vi "Hub_Connect to Laser_Dx.vi"() -> ()   [LabVIEW 2020]
uses:
  Anemometry/Anemometry Sub Vis/Globals/LDA_global.vi
panel:
  out "reference out":refnum<k7>
  in  "BSALaserCtrl.IBSALaser 2":refnum<k7>
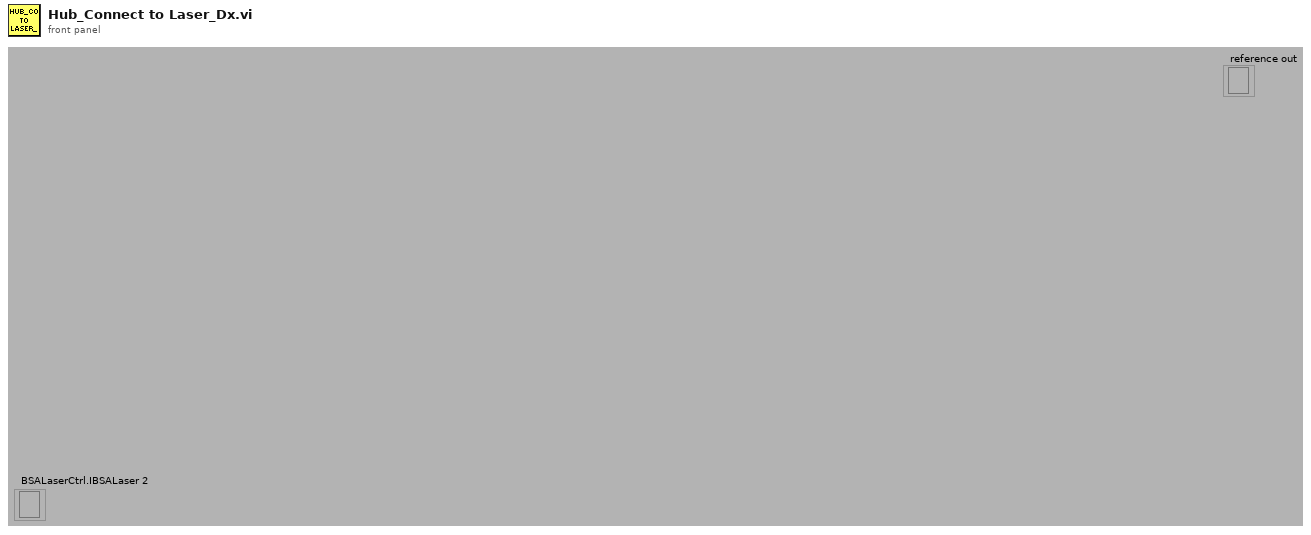
[diagram p1: front panel]
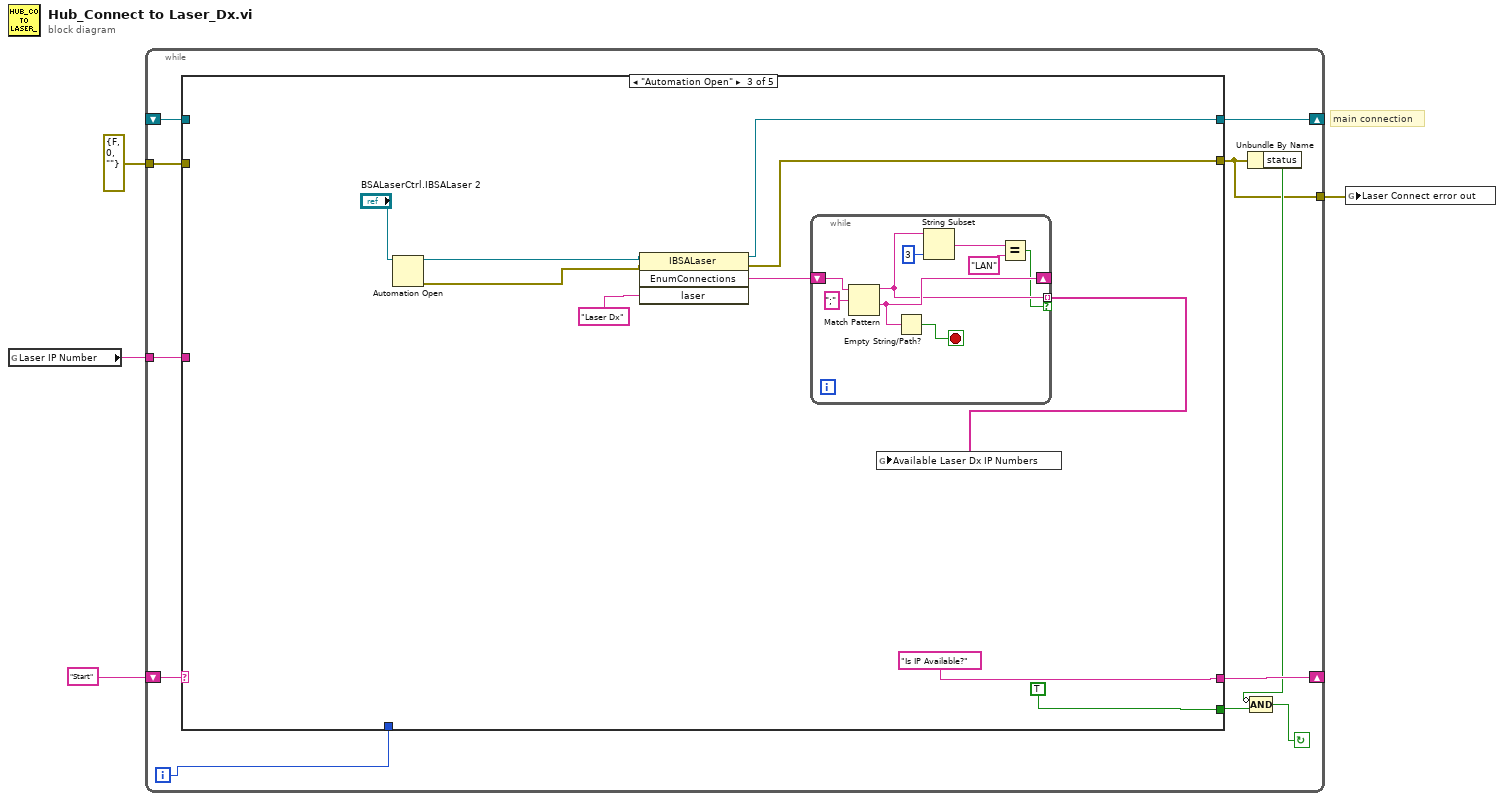
[diagram p0: block diagram]
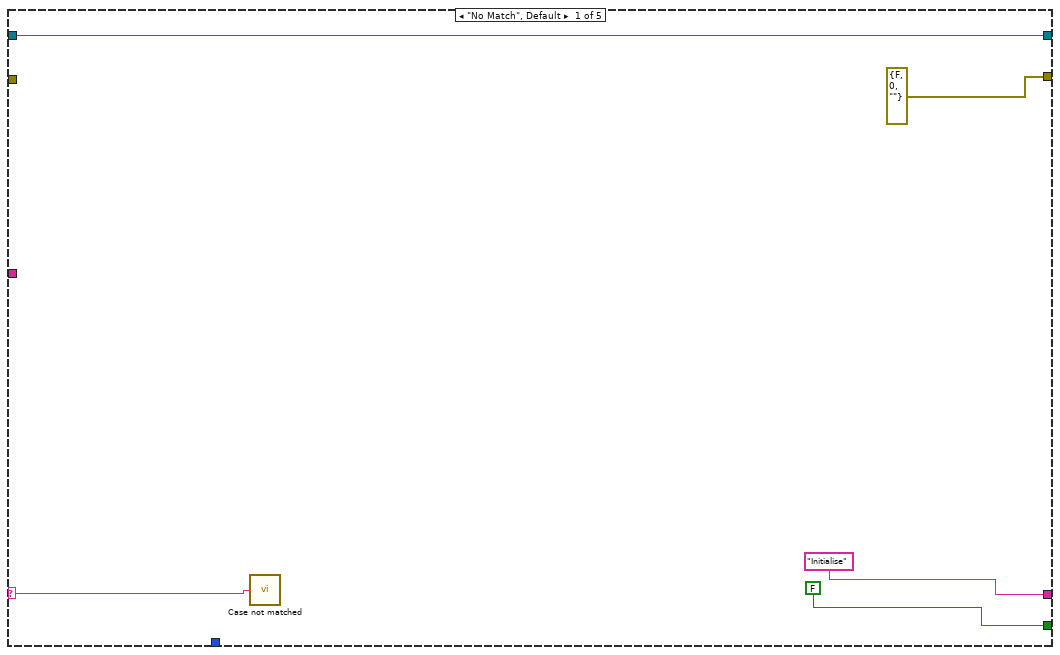
[diagram p2: hidden frame]
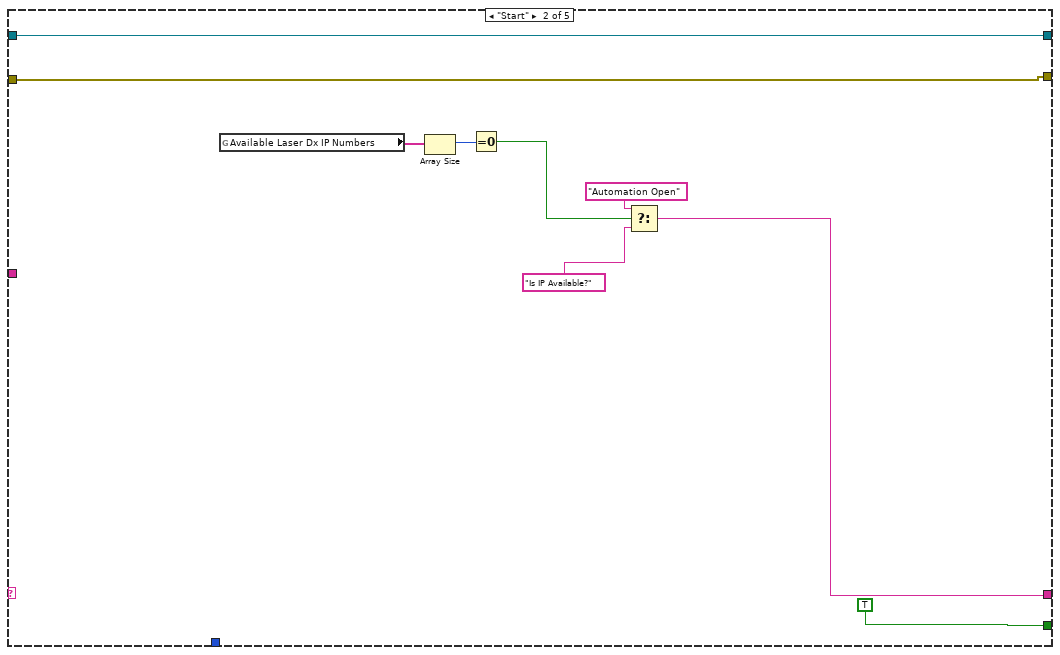
[diagram p3: hidden frame]
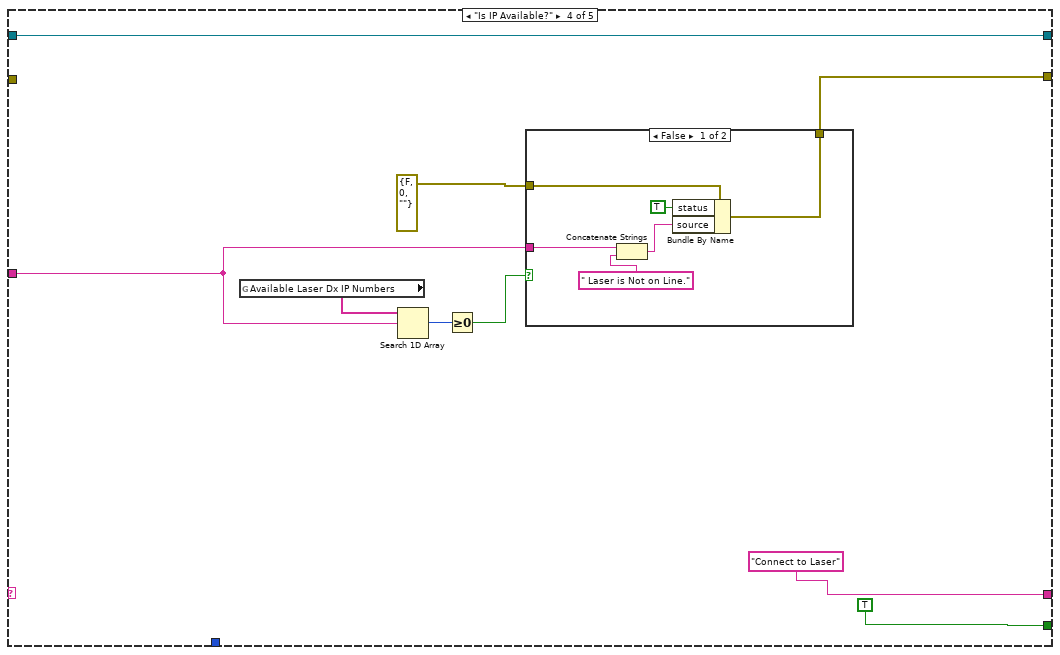
[diagram p4: hidden frame]
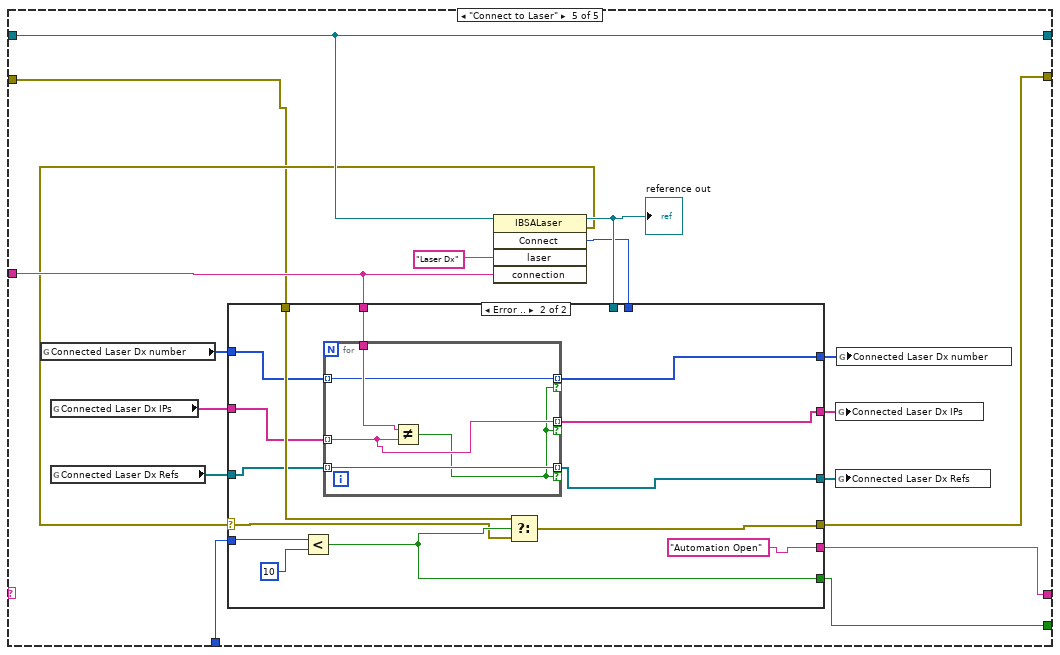
[diagram p6: hidden frame]
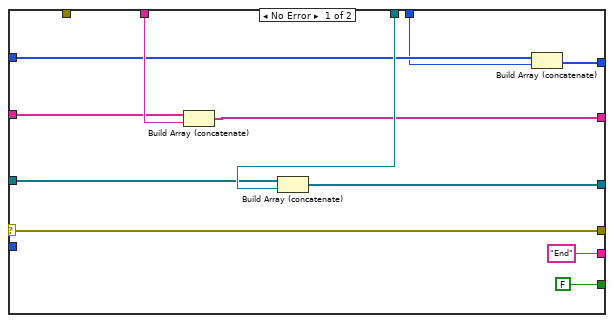
[diagram p7: hidden frame]
diagram:
  # "main connection"
  n1 = global read "LDA_global.vi" "Laser IP Number"() -> (w3:string)
  n2 = while {
    shift-left: "Start" -> [w14]
    shift-right: [w15] -> _
    shift-right: [w13] -> _
    shift-left: _ -> [w12]
    tunnel: w3 -> [w11]
    tunnel: [w7] -> w2
    tunnel: errorcluster {"status"=FALSE, "code"=0, "source"=""} ("error out") -> [w5]
    i -> [w6]
    stop <- w9 continue-if-true
    n3 = case shown="\"Automation Open\"" w14 {
      selector: w14 -> [w18 _ _ _ _]
      tunnel: [FALSE TRUE TRUE TRUE w74] -> w10
      tunnel: ["Initialise" w22 "Is IP Available?" "Connect to Laser" w73] -> w15
      tunnel: [w17 w26 w34 w54 w78] -> w13
      tunnel: w12 -> [w17 w26 _ w54 w78]
      tunnel: w11 -> [_ _ _ w49 w79]
      tunnel: [errorcluster {"status"=FALSE, "code"=0, "source"=""} ("error out") w21 w31 w52 w75] -> w7
      tunnel: w6 -> [_ _ _ _ w76]
      tunnel: w5 -> [_ w21 _ _ w72]
      frame "No Match", Default {
        n4 = call "Case not matched.vi"("Case Name not Matched"=w18) -> ()
      }
      frame "Start" {
        n5 = global read "LDA_global.vi" "Available Laser Dx IP Numbers"() -> (w28:string[])
        n6 = Array Size(array=w28) -> (size(s)=w27:i32)
        n7 = Equal To 0?(x=w27) -> (x = 0?=w25:bool)
        n8 = Select(t="Automation Open", s=w25, f="Is IP Available?") -> (s? t:f=w22:string)
      }
      frame "Automation Open" {
        n9 = Automation Open(Automation Refnum="BSALaserCtrl.IBSALaser 2") -> (Automation Refnum=w30:refnum<k7>, error out=w36:errorcluster)  [unwired: 3 in]
        n10 = invoke class="IBSALaser" method="EnumConnections"(reference=w30, error in=w36, "laser"="Laser Dx") -> (reference out=w34:refnum<k7>, error out=w31:errorcluster, "EnumConnections"=w38:string)  [unwired: 1 in, 1 out]
        n11 = while {
          shift-right: [w45] -> _
          shift-left: w38 -> [w47]
          tunnel: [w44] -> w33 mode=indexing if=w40
          stop <- w46 stop-if-true
          n12 = Match Pattern(string=w47, regular expression=";") -> (before substring=w44:string, after substring=w45:string)  [unwired: 1 in, 2 out]
          n13 = Empty String/Path?(string/path=w45) -> (empty?=w46:bool)
          n14 = String Subset(string=w44, length (rest)=3 ("length (rest)")) -> (substring=w42:string)  [unwired: 1 in]
          n15 = Equal?(x=w42, y="LAN") -> (x = y?=w40:bool)
        }
        n16 = global write "LDA_global.vi" "Available Laser Dx IP Numbers"(w33) -> ()
      }
      frame "Is IP Available?" {
        n17 = global read "LDA_global.vi" "Available Laser Dx IP Numbers"() -> (w56:string[])
        n18 = Search 1D Array(1D array=w56, element=w49) -> (index of element=w55:i32)  [unwired: 1 in]
        n19 = Greater Or Equal To 0?(x=w55) -> (x >= 0?=w53:bool)
        n20 = case shown="False" w53 {
          tunnel: [w62 w64] -> w52
          tunnel: errorcluster {"status"=FALSE, "code"=0, "source"=""} ("error out") -> [w63 w64]
          tunnel: w49 -> [w60 _]
          frame False {
            n21 = Concatenate Strings(w60, " Laser is Not on Line.") -> (w58:string)
            n22 = Bundle By Name(cluster=w63, "status"=TRUE, "source"=w58) -> (w62:errorcluster)
          }
          frame True {
          }
        }
      }
      frame "Connect to Laser" {
        n23 = global read "LDA_global.vi" "Connected Laser Dx number"() -> (w67:i64[])
        n24 = global read "LDA_global.vi" "Connected Laser Dx IPs"() -> (w71:string[])
        n25 = global read "LDA_global.vi" "Connected Laser Dx Refs"() -> (w70:refnum<k7>[])
        n26 = invoke class="IBSALaser" method="Connect"(reference=w78, "laser"="Laser Dx", "connection"=w79) -> (reference out=w80:refnum<k7>, error out=w77:errorcluster, "Connect"=w66:i64)  [unwired: 2 in, 2 out]
        "reference out" <- w80
        n27 = case shown="Error .." w77 {
          selector: w77 -> [w91 w102]
          tunnel: w80 -> [w93 _]
          tunnel: w79 -> [w92 w100]
          tunnel: w76 -> [_ w106]
          tunnel: [w91 w101] -> w75
          tunnel: [FALSE w104] -> w74
          tunnel: ["End" "Automation Open"] -> w73
          tunnel: w72 -> [_ w103]
          tunnel: w71 -> [w88 w99]
          tunnel: w70 -> [w87 w96]
          tunnel: [w86 w98] -> w69
          tunnel: [w85 w97] -> w68
          tunnel: w67 -> [w84 w94]
          tunnel: w66 -> [w83 _]
          tunnel: [w82 w95] -> w65
          frame No Error {
            n28 = Build Array (concatenate)(w88, w92) -> (w86:string[])
            n29 = Build Array (concatenate)(w87, w93) -> (w85:refnum<k7>[])
            n30 = Build Array (concatenate)(w84, w83) -> (w82:i64[])
          }
          frame Error {
            n31 = Less?(x=w106, y=10) -> (x < y?=w104:bool)
            n32 = for {
              tunnel: w100 -> [w112]
              tunnel: w99 -> [w111] mode=indexing
              tunnel: [w111] -> w98 mode=indexing if=w108
              tunnel: [w110] -> w97 mode=indexing if=w108
              tunnel: w96 -> [w110] mode=indexing
              tunnel: [w109] -> w95 mode=indexing if=w108
              tunnel: w94 -> [w109] mode=indexing
              n33 = Not Equal?(x=w112, y=w111) -> (x != y?=w108:bool)
            }
            n34 = Select(t=w103, s=w104, f=w102) -> (s? t:f=w101:errorcluster)
          }
        }
        n35 = global write "LDA_global.vi" "Connected Laser Dx IPs"(w69) -> ()
        n36 = global write "LDA_global.vi" "Connected Laser Dx Refs"(w68) -> ()
        n37 = global write "LDA_global.vi" "Connected Laser Dx number"(w65) -> ()
      }
    }
    n38 = Unbundle By Name(w7) -> ("status"=w8:bool)
    n39 = Compound Arithmetic op=AND(invert w8, w10) -> (w9:bool)
  }
  n40 = global write "LDA_global.vi" "Laser Connect error out"(w2) -> ()
